vi "Build Type Graph.vi"(4 "Descend into DVRs? (F)":bool, 6 "Unbundlable root only? (F)":bool, 7 "OwningVI":refnum<vi>, 10 "Max Depth (12)":i32=12, 11 "Type":variant) -> (0 "error out":errorcluster, 3 "Type Graph":T1[](array[typedef]))   [LabVIEW 2020, in "TypeGraph.lvlib"]
uses:
  TypeGraph.lvlib
  Type Reflection Item.ctl
  <vilib>/Utility/Data Type/NI_Data Type.lvlib
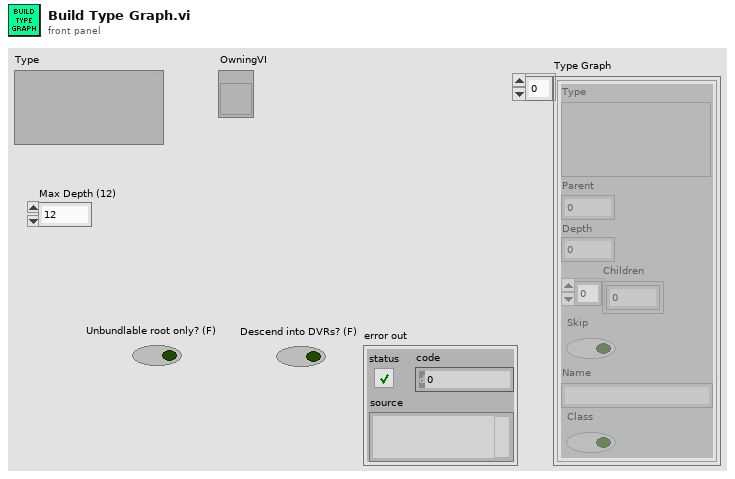
[diagram p1: front panel]
types:
  T1 = typedef "TypeGraph.lvlib/Type Reflection Item.ctl" = cluster{"Type":variant, "Parent":i32, "Depth":i32, "Children":i32[], "Skip":bool, "Name":string, "Class":bool}
  T2 = typedef "NI_Data Type.lvlib/Data Type.ctl" = enum8{"Invalid Type", "Void", "I8", "I16", "I32", "I64", "U8", "U16", "U32", "U64", "Single Float", "Double Float", "Extended Float", "Single Complex", "Double Complex", "Extended Complex", "Enum U8", "Enum U16", "Enum U32", "Enum U64", "Single Float With Unit", "Double Float With Unit", "Extended Float With Unit", "Single Complex with Unit", "Double Complex with Unit", "Extended Complex with Unit", "Boolean", "String", "Path", "Picture", "Tag", "Array", "Cluster", "Variant", "LV Variant", "Waveform", "Timestamp", "Digital Waveform", "Digital Data", "ExpressData", "Refnum", "External Data", "VI", "Poly VI", "LabVIEW Class Instance", "Fixed Point", "Set Collection", "Map Collection"}
  T3 = typedef "NI_Data Type.lvlib/Refnum Type.ctl" = enum16{"NotARefnum", "UnknownRefnum", "Generic", "Datalog", "ByteStream", "Device", "Occurence", "TCPNetConnection", "Auto", "Menu", "Imaq", "Hardware", "DataSocket", "Visa", "IVI", "UDPNetConnection", "Notifier", "Queue", "Irda", "EventReg", "DotNet", "UserEvent", "Callback", "UNUSED_EMPTY_POSITION", "BlueToothNetConnection", "LVObjApp", "LVObjVI", "LVObjUnknown", "GenericClass", "UserDefinedRefnumTag", "DataValue", "RT FIFO", "TDMS File", "PythonSessionRefnum"}
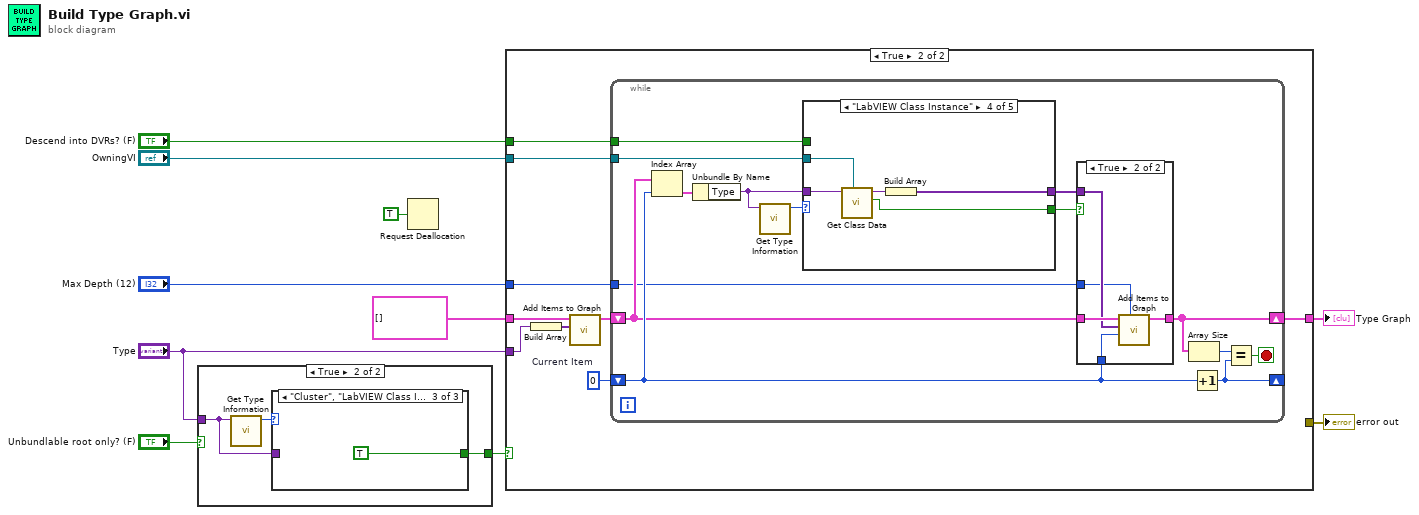
[diagram p0: block diagram]
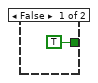
[diagram p2: hidden frame]
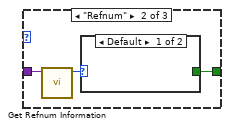
[diagram p4: hidden frame]
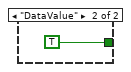
[diagram p5: hidden frame]
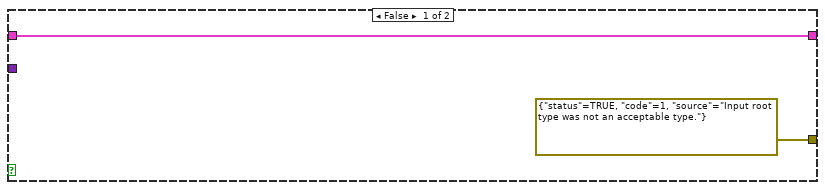
[diagram p6: hidden frame]
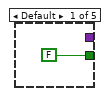
[diagram p7: hidden frame]
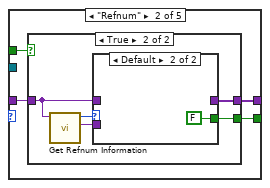
[diagram p8: hidden frame]
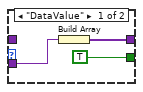
[diagram p10: hidden frame]
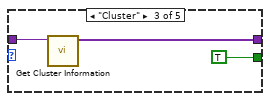
[diagram p11: hidden frame]
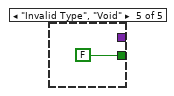
[diagram p12: hidden frame]
diagram:
  n1 = case shown="True" "Unbundlable root only? (F)" {
    tunnel: [TRUE w13] -> w10
    tunnel: "Type" -> [_ w12]
    frame False {
    }
    frame True {
      n2 = call <vilib>:"Get Type Information.vi"("variant"=w12) -> ("type"=w14:T2)  [unwired: 6 in, 4 out]
      n3 = case shown="\"Cluster\", \"LabVIEW Class Instance\"" w14 {
        tunnel: w12 -> [_ w17 _]
        tunnel: [_ w15 TRUE] -> w13
        frame Default {
        }
        frame "Refnum" {
          n4 = call <vilib>:"Get Refnum Information.vi"("variant"=w17) -> ("reference type"=w16:T3)  [unwired: 7 in, 3 out]
          n5 = case shown="Default" w16 {
            tunnel: [_ TRUE] -> w15
            frame Default {
            }
            frame "DataValue" {
            }
          }
        }
        frame "Cluster", "LabVIEW Class Instance" {
        }
      }
    }
  }
  n6 = Request Deallocation(TRUE ("flag")) -> ()
  n7 = case shown="True" w10 {
    tunnel: "Type" -> [_ w28]
    tunnel: T1[] [] ("Item Graph") -> [w20 w30]
    tunnel: [w20 w26] -> w8
    tunnel: [errorcluster {"status"=TRUE, "code"=1, "source"="Input root type was not an acceptable type."} ("error constant") _] -> w7
    tunnel: "OwningVI" -> [_ w24]
    tunnel: "Max Depth (12)" -> [_ w23]
    tunnel: "Descend into DVRs? (F)" -> [_ w22]
    frame False {
    }
    frame True {
      w27 = 0  # Current Item
      n8 = Build Array(w28) -> (w25:variant[])
      n9 = call "Add Items to Graph.vi"("Items"=w25, "Graph In"=w30) -> ("Graph"=w29:T1[])  [unwired: 9 in]
      n10 = while {
        shift-right: [w41] -> w26
        shift-left: w29 -> [w39]
        shift-right: [w43] -> _
        shift-left: w27 -> [w40]
        tunnel: w24 -> [w35]
        tunnel: w23 -> [w32]
        tunnel: w22 -> [w31]
        stop <- w42 stop-if-true
        n11 = Index Array(array=w39, index=w40) -> (element=w38:T1)
        n12 = Unbundle By Name(w38) -> ("Type"=w36:variant)
        n13 = call <vilib>:"Get Type Information.vi"("variant"=w36) -> ("type"=w37:T2)  [unwired: 6 in, 4 out]
        n14 = case shown="\"LabVIEW Class Instance\"" w37 {
          tunnel: w36 -> [_ w49 w61 w66 _]
          tunnel: w35 -> [_ _ _ w65 _]
          tunnel: [FALSE w47 TRUE w62 FALSE] -> w34
          tunnel: [_ w48 w60 w63 _] -> w33
          tunnel: w31 -> [_ w46 _ _ _]
          frame Default {
          }
          frame "Refnum" {
            n15 = case shown="True" w46 {
              tunnel: w49 -> [_ w53]
              tunnel: [_ w51] -> w48
              tunnel: [_ w50] -> w47
              frame False {
              }
              frame True {
                n16 = call <vilib>:"Get Refnum Information.vi"("variant"=w53) -> ("strict type"=w52:variant, "reference type"=w54:T3)  [unwired: 7 in, 2 out]
                n17 = case shown="Default" w54 {
                  tunnel: w53 -> [_ _]
                  tunnel: w52 -> [w57 _]
                  tunnel: [w56 _] -> w51
                  tunnel: [TRUE FALSE] -> w50
                  frame "DataValue" {
                    n18 = Build Array(w57) -> (w56:variant[])
                  }
                  frame Default {
                  }
                }
              }
            }
          }
          frame "Cluster" {
            n19 = call <vilib>:"Get Cluster Information.vi"("variant"=w61) -> ("cluster elements"=w60:variant[])  [unwired: 9 in, 1 out]
          }
          frame "LabVIEW Class Instance" {
            n20 = call "Get Class Data.vi"("OwningVI"=w65, "Class"=w66) -> ("Can Access Members?"=w62:bool, "Class Data"=w64:variant)  [unwired: 8 in]
            n21 = Build Array(w64) -> (w63:variant[])
          }
          frame "Invalid Type", "Void" {
          }
        }
        n22 = case shown="True" w34 {
          tunnel: w39 -> [w68 w73]
          tunnel: [w68 w72] -> w41
          tunnel: w40 -> [_ w71]
          tunnel: w33 -> [_ w70]
          tunnel: w32 -> [_ w69]
          frame False {
          }
          frame True {
            n23 = call "Add Items to Graph.vi"("Depth Limit (12)"=w69, "Parent Index (None)"=w71, "Items"=w70, "Graph In"=w73) -> ("Graph"=w72:T1[])  [unwired: 7 in]
          }
        }
        n24 = Array Size(array=w41) -> (size(s)=w44:i32)
        n25 = Increment(x=w40) -> (x+1=w43:i32)
        n26 = Equal?(x=w44, y=w43) -> (x = y?=w42:bool)
      }
    }
  }
  "Type Graph" <- w8
  "error out" <- w7
